vi "Escritura.vi"(1 "error out":errorcluster) -> (0 "String":string)   [LabVIEW 2015]
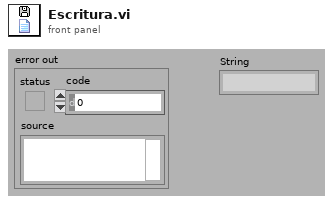
[diagram p1: front panel]
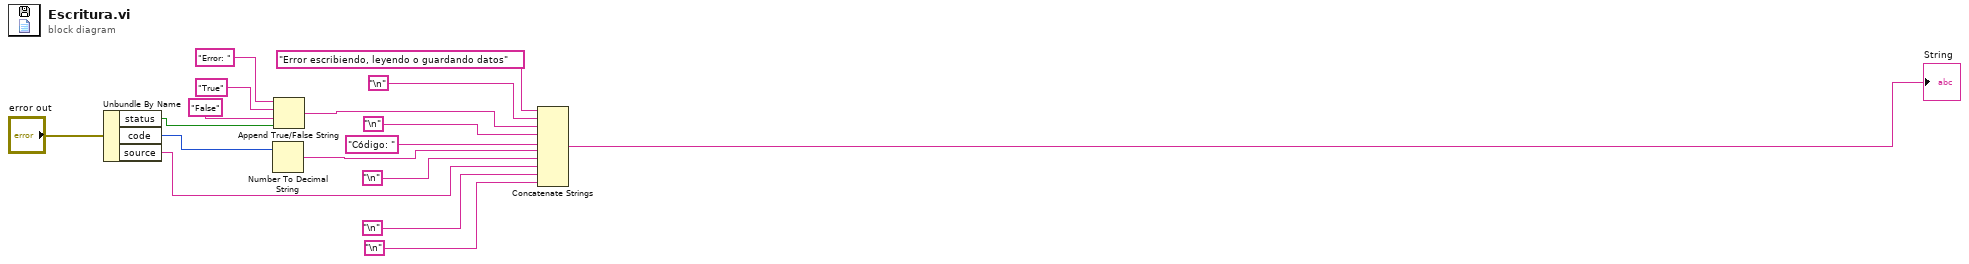
[diagram p0: block diagram]
diagram:
  n1 = Unbundle By Name("error out") -> ("status"=w5:bool, "code"=w6:i32, "source"=w14:string)
  n2 = Number To Decimal String(number=w6) -> (decimal integer string=w12:string)  [unwired: 1 out]
  n3 = Append True/False String(1:w5, 2:"False" ("false string"), 3:"True" ("true string"), 4:"Error: " ("string (\"\")")) -> (0:w9:string)
  n4 = Concatenate Strings("Error escribiendo, leyendo o guardando datos", "\n", w9, "\n", "Código: " ("string (\"\")"), w12, "\n", w14, "\n", "\n") -> (→"String":string)
